vi "Coord window-Handle mouse wheel.vi"(11 "Delta":i32) -> ()   [LabVIEW 2013]
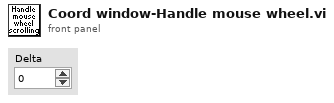
[diagram p1: front panel]
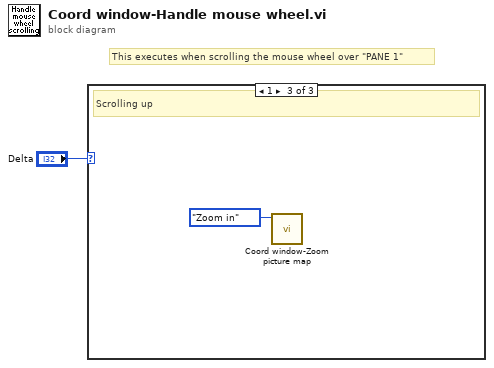
[diagram p0: block diagram]
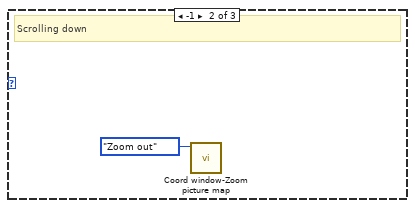
[diagram p3: hidden frame]
diagram:
  # "This executes when scrolling the mouse wheel over \"PANE 1\""
  n1 = case shown="1" "Delta" {
    frame Default {
    }
    frame -1 {
      # "Scrolling down"
      n2 = call "Coord window-Zoom picture map.vi"("Function"=enum16{"Zoom in", "Zoom out"}."Zoom out") -> ()  [unwired: 11 in]
    }
    frame 1 {
      # "Scrolling up"
      n3 = call "Coord window-Zoom picture map.vi"("Function"=enum16{"Zoom in", "Zoom out"}."Zoom in") -> ()  [unwired: 11 in]
    }
  }
